vi "Test.vi"() -> ()   [LabVIEW 2012, in "Universal Power Meter.lvlib" / "Yokogawa WT2X0.lvlib" / "Yokogawa WT2X0.lvclass"]
uses:
  Yokogawa WT2X0.lvclass
panel:
  out "subarray":string[](array[string])
  out "x+1":i32
  out "Array 2":string[][](array[string])
  out "Array":string[][](array[string])
  out "error out":errorcluster
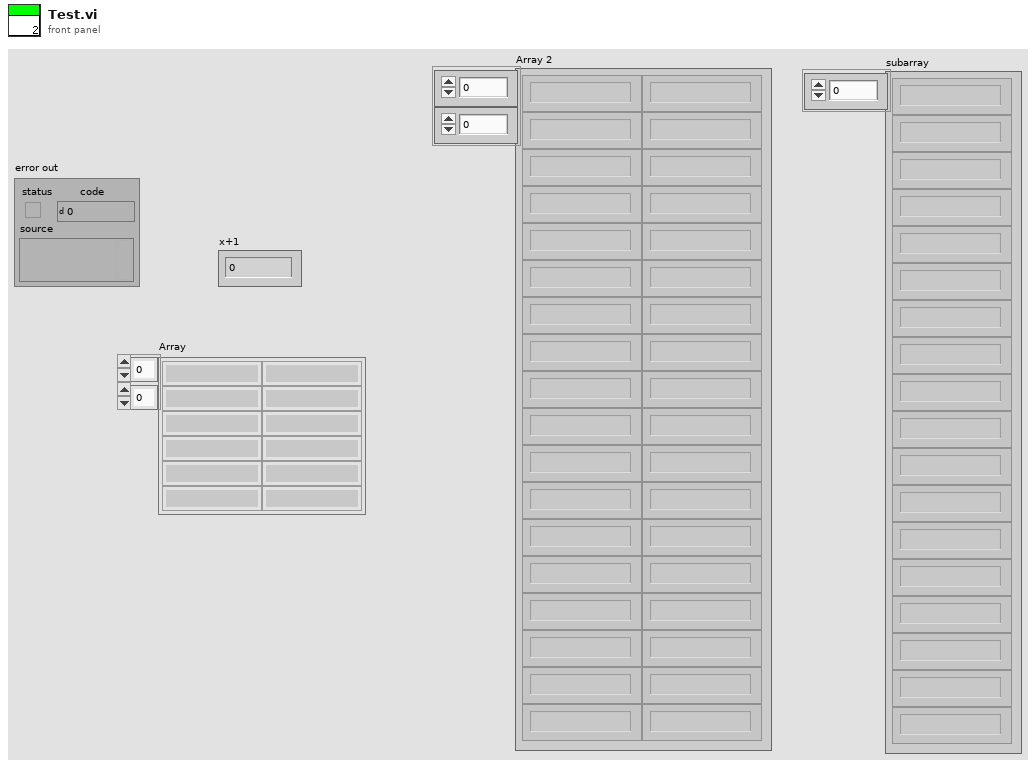
[diagram p1: front panel]
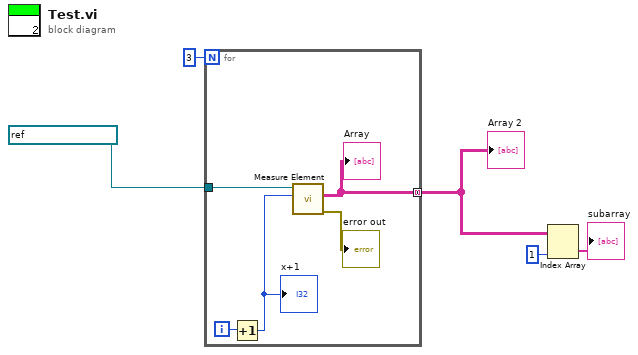
[diagram p0: block diagram]
diagram:
  n1 = for {
    N: 3 -> [_]
    tunnel: refnum<visa-resource-name> "GPIB0::1::INSTR" ("VISA resource name") -> [w10]
    tunnel: [w6] -> w3 mode=concatenating
    i -> [w9]
    n2 = Increment(x=w9) -> (x+1=w8:i32)
    "x+1" <- w8
    n3 = call "Measure Element.vi"("Element (1: Element 1)"=w8, "VISA resource name"=w10) -> ("error out"=→"error out":errorcluster, "Array"=w6:string[][])  [unwired: 7 in, 1 out]
    "Array" <- w6
  }
  "Array 2" <- w3
  n4 = Index Array(array=w3, index (col)=1 ("disabled index (col)")) -> (element=→"subarray":string[])  [unwired: 1 in]
